vi "IF2_TagBuffer.vi"(7 "Action":enum16{"Init", "WriteTagData", "ReadTagData"}(ring), 8 "error in":errorcluster, 11 "TagData in":cluster{"TagCode":string, "FirstSeemUs":u64}) -> (0 "error out":errorcluster, 3 "TagData out":cluster{"TagCode":string, "FirstSeemUs":u64}[](array[cluster]))   [LabVIEW 2015, in "IF2_Reader.lvlib"]
uses:
  IF2_Reader.lvlib
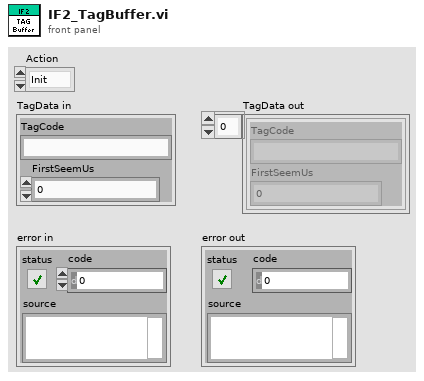
[diagram p1: front panel]
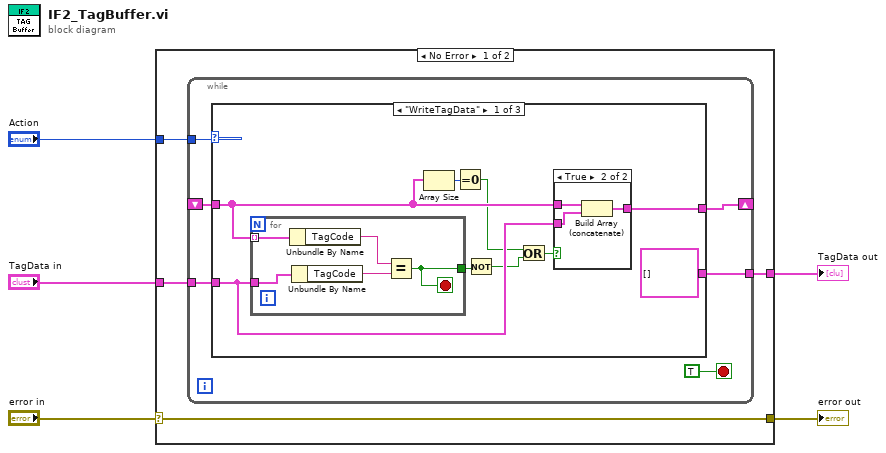
[diagram p0: block diagram]
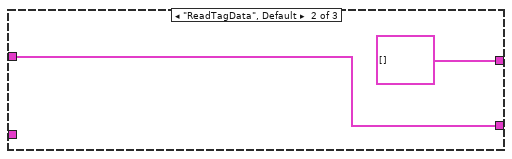
[diagram p3: hidden frame]
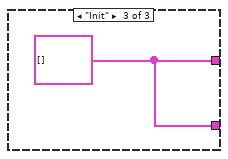
[diagram p4: hidden frame]
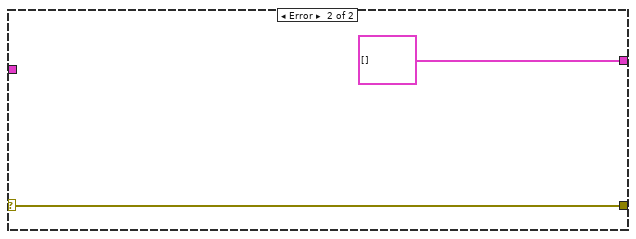
[diagram p5: hidden frame]
diagram:
  n1 = case shown="No Error" "error in" {
    selector: "error in" -> [w6 w37]
    tunnel: "Action" -> [w9 _]
    tunnel: "TagData in" -> [w8 _]
    tunnel: [w7 cluster{"TagCode":string, "FirstSeemUs":u64}[] []] -> w3
    tunnel: [w6 w37] -> w5
    frame No Error {
      n2 = while {
        tunnel: w9 -> [w15]
        tunnel: w8 -> [w12]
        shift-right: [w11] -> _
        shift-left: _ -> [w14]
        tunnel: [w10] -> w7
        stop <- TRUE stop-if-true
        n3 = case shown="\"WriteTagData\"" w15 {
          tunnel: w14 -> [w19 w34 _]
          tunnel: w12 -> [w22 _ _]
          tunnel: [w24 cluster{"TagCode":string, "FirstSeemUs":u64}[] [] w36] -> w11
          tunnel: [cluster{"TagCode":string, "FirstSeemUs":u64}[] [] w34 w36] -> w10
          frame "WriteTagData" {
            n4 = for {
              tunnel: w22 -> [w29]
              tunnel: w19 -> [w32] mode=indexing
              tunnel: [w30] -> w18
              stop <- w30 stop-if-true
              n5 = Unbundle By Name(w32) -> ("TagCode"=w33:string)
              n6 = Unbundle By Name(w29) -> ("TagCode"=w31:string)
              n7 = Equal?(x=w33, y=w31) -> (x = y?=w30:bool)
            }
            n8 = Array Size(array=w19) -> (size(s)=w20:i32)
            n9 = Equal To 0?(x=w20) -> (x = 0?=w17:bool)
            n10 = Not(x=w18) -> (.not. x?=w16:bool)
            n11 = Or(x=w17, y=w16) -> (x .or. y?=w21:bool)
            n12 = case shown="True" w21 {
              tunnel: w19 -> [w25 w28]
              tunnel: w22 -> [_ w27]
              tunnel: [w25 w26] -> w24
              frame False {
              }
              frame True {
                n13 = Build Array (concatenate)(w28, w27) -> (w26:cluster{"TagCode":string, "FirstSeemUs":u64}[])
              }
            }
          }
          frame "ReadTagData", Default {
          }
          frame "Init" {
            w36 = cluster{"TagCode":string, "FirstSeemUs":u64}[] []
          }
        }
      }
    }
    frame Error {
    }
  }
  "TagData out" <- w3
  "error out" <- w5
